vi "读取数据库.vi"(7 "condition":string, 8 "error in (no error)":errorcluster caption="错误输入（无错误）", 9 "database":string="database1.mdb", 10 "显示项":string[](array[string]), 11 "组合框":string(combo)) -> (0 "error out":errorcluster caption="错误输出", 1 "columns":string[](array[string]), 2 "data":variant[][](array[variant]), 3 "表格":string[][](table))   [LabVIEW 2016, in "数据查询.lvlib"]
uses:
  <vilib>/addons/database/Connection.llb/DB Tools Open Connec (String).vi
  <vilib>/addons/database/_DB Variant To Data/Database Variant To Data.xnode
  <vilib>/addons/database/NI_Database_API.lvlib
  database/Access/Access Lib.lvlib
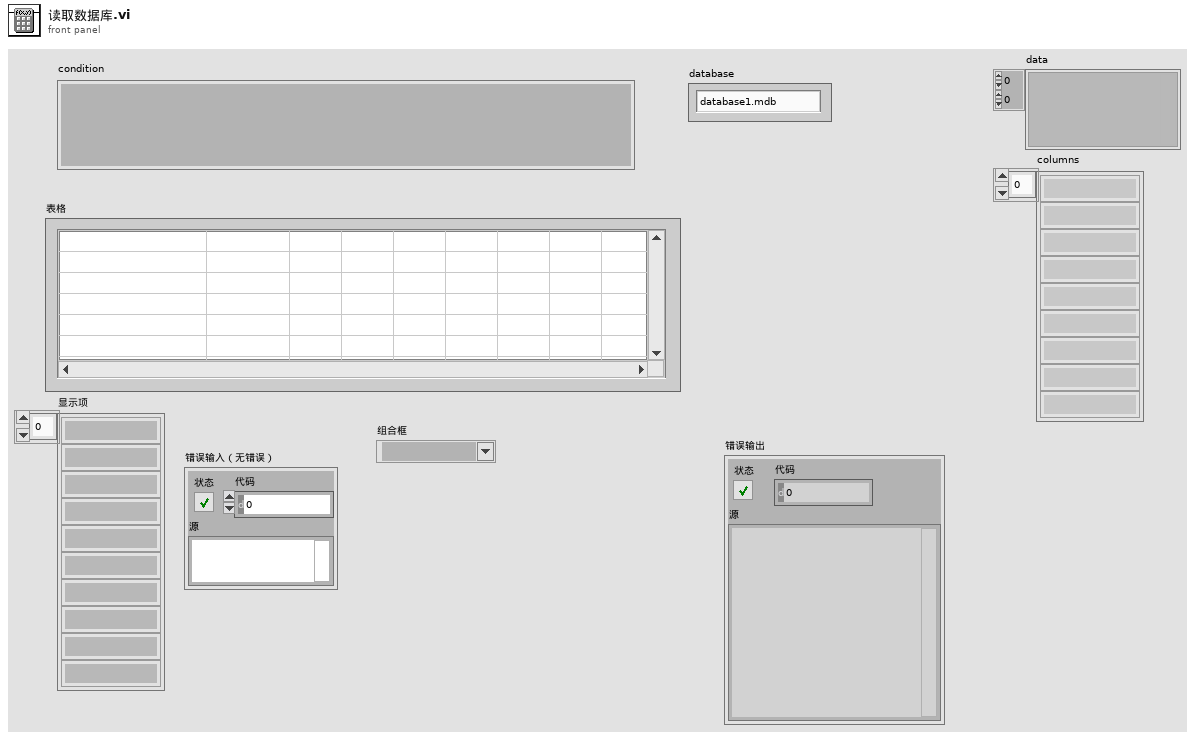
[diagram p1: front panel]
types:
  T1 = typedef "NI_Database_API.lvlib/Conn ObjectReference.ctl" = refnum<k1>
  T2 = typedef "NI_Database_API.lvlib/DB Tools DataTypes.ctl" = enum16{"String", "Long (I32)", "Single (SGL)", "Double (DBL)", "Date/Time", "Binary"}
  T3 = cluster{"name":string, "database data type":T2, "defined size":i32}[]
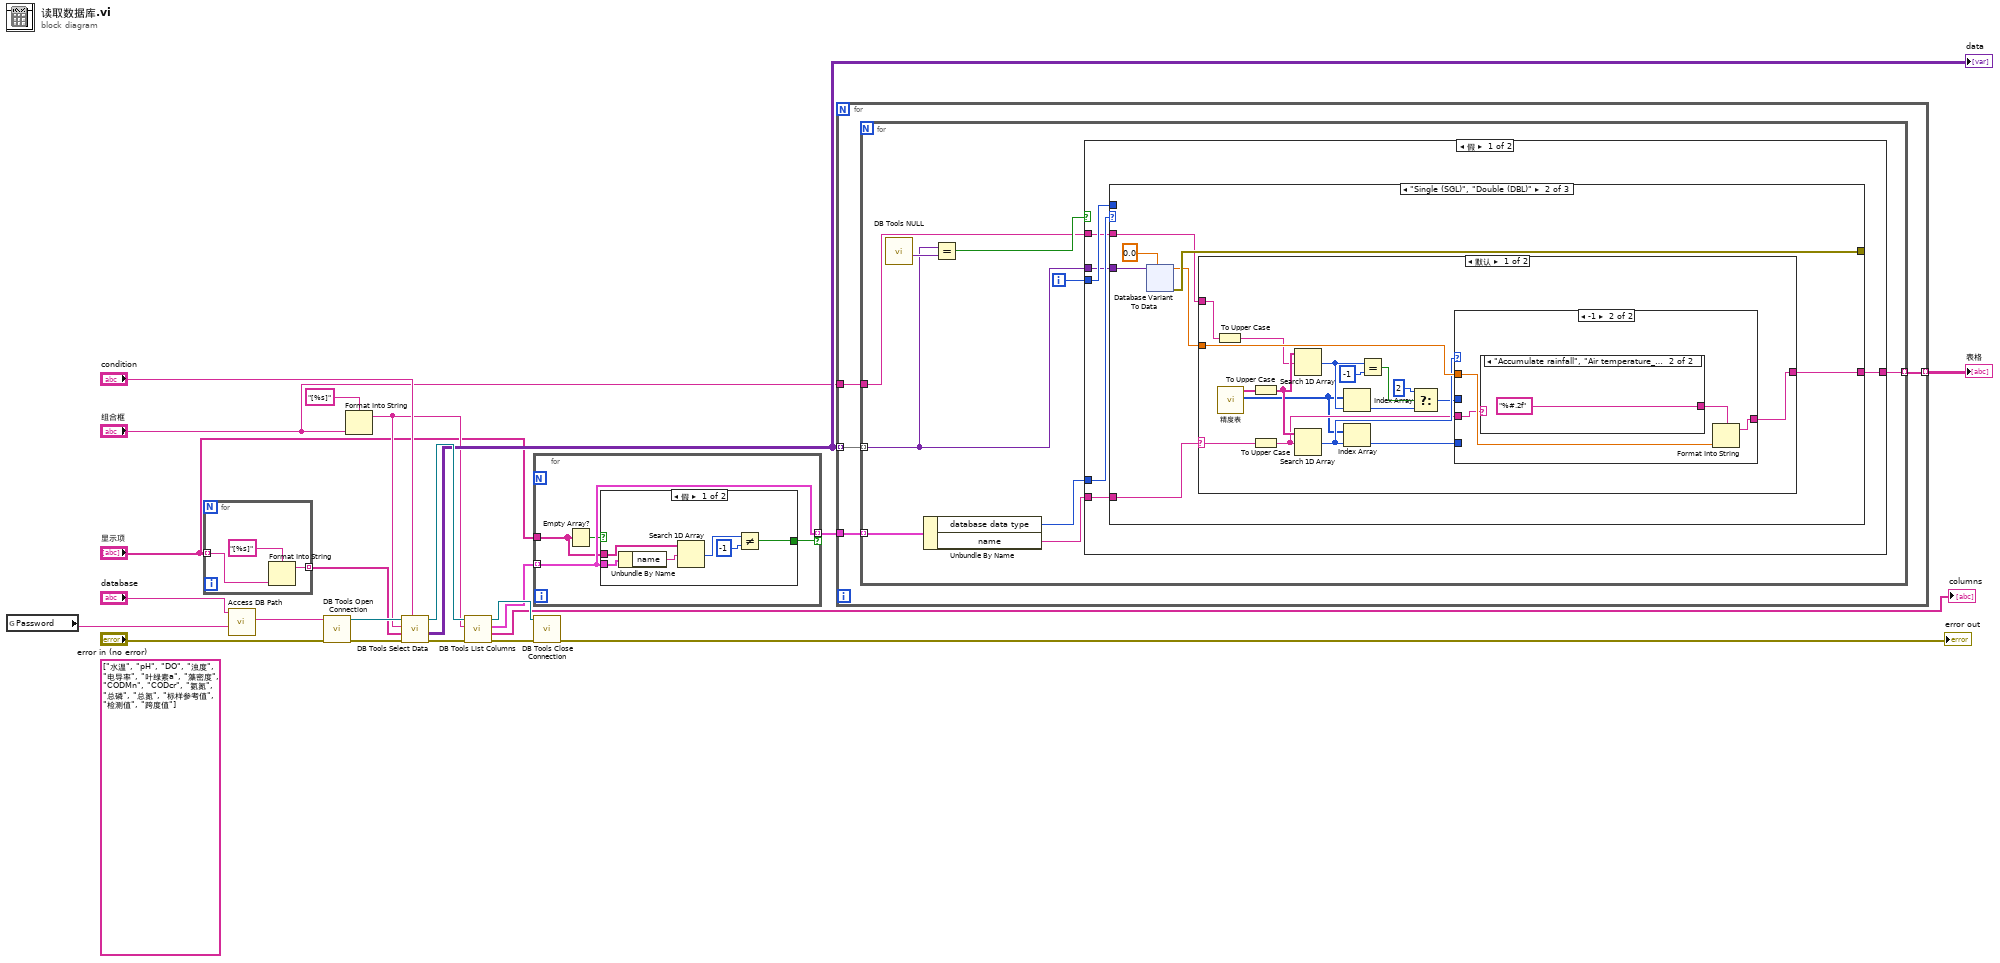
[diagram p0: block diagram]
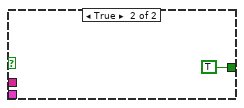
[diagram p2: hidden frame]
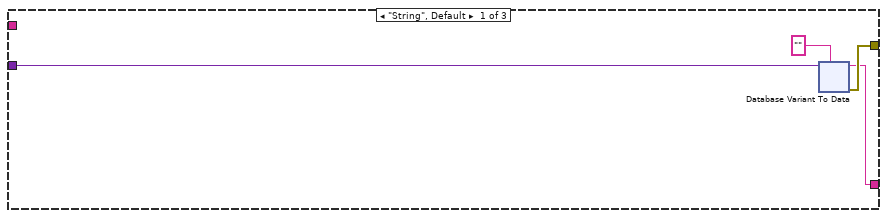
[diagram p3: hidden frame]
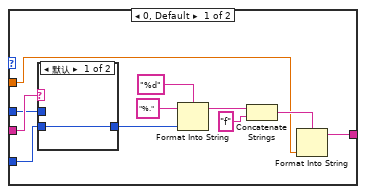
[diagram p4: hidden frame]
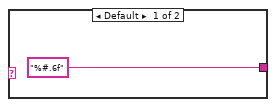
[diagram p6: hidden frame]
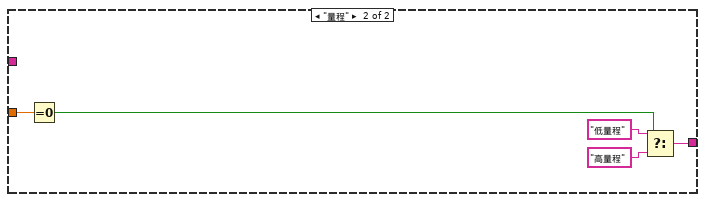
[diagram p7: hidden frame]
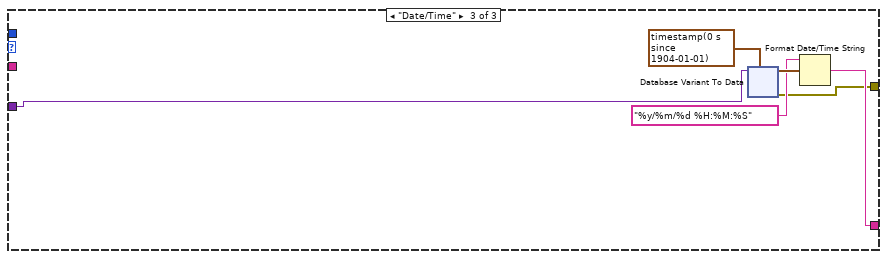
[diagram p8: hidden frame]
diagram:
  (unwired) string[] ["水温", "pH", "DO", "浊度", "电导率", "叶绿素a", "藻密度", "CODMn", "CODcr", "氨氮", "总磷", "总氮", "标样参考值", "检测值", "跨度值"]
  n1 = global read "全局变量.vi" "Password"() -> (w1:string)
  n2 = for {
    tunnel: "显示项" -> [w25] mode=indexing
    tunnel: [w24] -> w2 mode=indexing
    n3 = Format Into String(format string="[%s]" ("格式字符串"), w25) -> (resulting string=w24:string)  [unwired: 2 in, 1 out]
  }
  n4 = call "Access DB Path.vi"("Password"=w1, "database"="database") -> ("Connection information"=w4:string)  [unwired: 8 in, 1 out]
  n5 = call-poly <vilib>:"DB Tools Open Connection.vi"("error in (no error)"="error in (no error)", "connection information"=w4) -> ("error out"=w21:errorcluster, "connection reference"=w22:T1)  [unwired: 6 in]
  n6 = Format Into String(format string="[%s]" ("格式字符串"), "组合框") -> (resulting string=w8:string)  [unwired: 2 in, 1 out]
  n7 = call <vilib>:"DB Tools Select Data.vi"("condition"="condition", "error in (no error)"=w21, "columns"=w2, "table"=w8, "connection reference"=w22) -> ("error out"=w20:errorcluster, "data"=w13:variant[][], "connection reference out"=w17:T1)  [unwired: 1 in]
  "data" <- w13
  n8 = call <vilib>:"DB Tools List Columns.vi"("error in (no error)"=w20, "table"=w8, "connection reference"=w17) -> ("error out"=w14:errorcluster, "columns"=→"columns":string[], "column information"=w10:T3, "connection reference out"=w15:T1)  [unwired: 1 in]
  n9 = for {
    tunnel: w10 -> [w28] mode=indexing
    tunnel: "显示项" -> [w27]
    tunnel: [w28] -> w9 mode=indexing if=w29
    n10 = Empty Array?(array=w27) -> (empty?=w26:bool)
    n11 = case shown="假" w26 {
      tunnel: [w32 TRUE] -> w29
      tunnel: w28 -> [w31 _]
      tunnel: w27 -> [w30 _]
      frame False {
        n12 = Unbundle By Name(w31) -> ("name"=w33:string)
        n13 = Search 1D Array(1D array=w30, element=w33) -> (index of element=w35:i32)  [unwired: 1 in]
        n14 = Not Equal?(x=w35, y=-1) -> (x != y?=w32:bool)
      }
      frame True {
      }
    }
  }
  n15 = call <vilib>:"DB Tools Close Connection.vi"("error in (no error)"=w14, "connection reference"=w15) -> ("error out"=→"error out":errorcluster)  [unwired: 5 in]
  n16 = for {
    tunnel: w13 -> [w40] mode=indexing
    tunnel: w9 -> [w39]
    tunnel: [w38] -> w12 mode=indexing
    tunnel: "组合框" -> [w37]
    n17 = for {
      tunnel: w40 -> [w45] mode=indexing
      tunnel: w39 -> [w49] mode=indexing
      tunnel: [w47] -> w38 mode=indexing
      tunnel: w37 -> [w43]
      i -> [w48]
      n18 = call <vilib>:"DB Tools NULL.vi"() -> ("NULL"=w46:variant)  [unwired: 10 in, 1 out]
      n19 = Unbundle By Name(w49) -> ("database data type"=w42:T2, "name"=w41:string)
      n20 = Equal?(x=w45, y=w46) -> (x = y?=w44:bool)
      n21 = case shown="假" w44 {
        tunnel: w42 -> [w55 _]
        tunnel: w48 -> [w54 _]
        tunnel: [w53 _] -> w47
        tunnel: w41 -> [w52 _]
        tunnel: w45 -> [w51 _]
        tunnel: w43 -> [w50 _]
        frame False {
          n22 = case shown="\"Single (SGL)\", \"Double (DBL)\"" w55 {
            tunnel: w51 -> [w59 w96 w177]
            tunnel: [w56 w97 w173] -> w53
            tunnel: w54 -> [_ _ _]
            tunnel: [w57 w98 w172] -> _
            tunnel: w52 -> [_ w95 _]
            tunnel: w50 -> [_ w92 _]
            frame "String", Default {
              n23 = xnode "Database Variant To Data"("database variant"=w59, "type"="") -> ("data"=w56:string, "error out"=w57:errorcluster)  [unwired: 1 in]
            }
            frame "Single (SGL)", "Double (DBL)" {
              n24 = xnode "Database Variant To Data"("database variant"=w96, "type"=0.0) -> ("data"=w93:dbl, "error out"=w98:errorcluster)  [unwired: 1 in]
              n25 = case shown="默认" w95 {
                selector: w95 -> [w113 _]
                tunnel: w93 -> [w115 w139]
                tunnel: [w114 w135] -> w97
                tunnel: w92 -> [w111 _]
                frame Default {
                  n26 = To Upper Case(1:w111) -> (0:w108:string)
                  n27 = call "精度表.vi"() -> ("精度"=w99:i32[], "参数"=w100:string[])  [unwired: 10 in]
                  n28 = To Upper Case(1:w100) -> (0:w109:string[])
                  n29 = To Upper Case(1:w113) -> (0:w107:string)
                  n30 = Search 1D Array(1D array=w109, element=w108) -> (index of element=w106:i32)  [unwired: 1 in]
                  n31 = Search 1D Array(1D array=w109, element=w107) -> (index of element=w112:i32)  [unwired: 1 in]
                  n32 = Index Array(array=w99, index=w106) -> (element=w103:i32)
                  n33 = Index Array(array=w99, index=w112) -> (element=w110:i32)
                  n34 = Equal?(x=w106, y=-1) -> (x = y?=w104:bool)
                  n35 = Select(t=2, s=w104, f=w103) -> (s? t:f=w102:i32)
                  n36 = case shown="-1" w112 {
                    tunnel: w115 -> [w120 w132]
                    tunnel: [w118 w131] -> w114
                    tunnel: w107 -> [w119 w129]
                    tunnel: w102 -> [w117 _]
                    tunnel: w110 -> [w116 _]
                    frame 0, Default {
                      n37 = case shown="默认" w119 {
                        tunnel: [w127 w128] -> w126
                        tunnel: w117 -> [_ w128]
                        tunnel: w116 -> [w127 _]
                        frame Default {
                        }
                        frame "检测值" {
                        }
                      }
                      n38 = Format Into String(format string="%d" ("格式字符串"), initial string="%." ("初始字符串"), w126) -> (resulting string=w124:string)  [unwired: 1 in, 1 out]
                      n39 = Concatenate Strings(w124, "f" ("格式字符串")) -> (w122:string)
                      n40 = Format Into String(format string=w122, w120) -> (resulting string=w118:string)  [unwired: 2 in, 1 out]
                    }
                    frame -1 {
                      n41 = case shown="\"Accumulate rainfall\", \"Air temperature_℃\", \"Barometric pressure_B\", \"Humidity\", \"Wind direction_degrees True\", \"Wind speed_m/s\", \"电压\", \"湿度\", \"温度\"" w129 {
                        tunnel: ["%#.6f" ("格式字符串") "%#.2f" ("格式字符串")] -> w130
                        frame Default {
                        }
                        frame "Accumulate rainfall", "Air temperature_℃", "Barometric pressure_B", "Humidity", "Wind direction_degrees True", "Wind speed_m/s", "电压", "湿度", "温度" {
                        }
                      }
                      n42 = Format Into String(format string=w130, w132) -> (resulting string=w131:string)  [unwired: 2 in, 1 out]
                    }
                  }
                }
                frame "量程" {
                  n43 = Equal To 0?(x=w139) -> (x = 0?=w138:bool)
                  n44 = Select(t="低量程" ("格式字符串"), s=w138, f="高量程" ("格式字符串")) -> (s? t:f=w135:string)
                }
              }
            }
            frame "Date/Time" {
              n45 = xnode "Database Variant To Data"("database variant"=w177, "type"=timestamp(0 s since 1904-01-01) ("当前时间")) -> ("data"=w176:timestamp, "error out"=w172:errorcluster)  [unwired: 1 in]
              n46 = Format Date/Time String(time format string (%c)="%y/%m/%d %H:%M:%S" ("时间格式字符串(%c)"), seconds (now)=w176) -> (date/time string=w173:string)  [unwired: 1 in]
            }
          }
        }
        frame True {
        }
      }
    }
  }
  "表格" <- w12
